vi "Configure Multi Eval Meas Limit ACLR Test Tolerance.vi"(7 "Tolerance 30-40 (5.0)":dbl=5.0 format="%^.3e", 8 "error in (no error)":errorcluster, 9 "Tolerance 23-30 (4.6)":dbl=4.6 format="%^.3e", 10 "Instance (1)":T1=1, 11 "VISA resource name":refnum<visa-resource-name>) -> (0 "error out":errorcluster, 3 "VISA resource name out":refnum<visa-resource-name>)   [LabVIEW 2020, in "Rohde&Schwarz CMXP NR FR2 Measurement.lvlib"]
doc: "Defines the test tolerance for relative ACLR limits, depending on the carrier frequency.\n\nAttribute:\nRSCMXPNRFR2M_ATTR_MULTI_EVAL_MEASUREMENT_LIMIT_ACLR_TEST_TOLERANCE\n\nRemote-control command:\nCONFigure:NRMMw:MEAS<i>:MEValuation:LIMit:ACLR:ATTolerance"
uses:
  <instrlib>/Rohde&Schwarz CMXP NR FR2 Measurement/Rohde&Schwarz CMXP NR FR2 Measurement.lvlib
  <instrlib>/Rohde&Schwarz CMXP NR FR2 Measurement/Private/_Instance.ctl
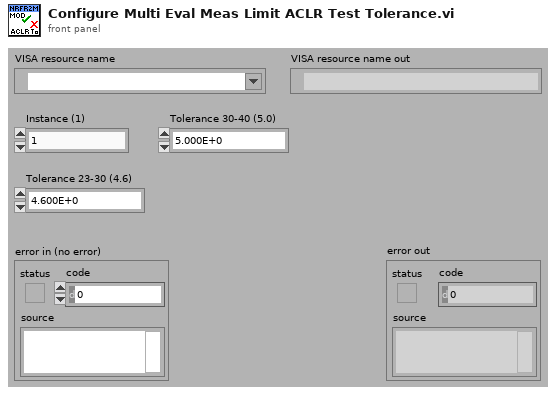
[diagram p1: front panel]
types:
  T1 = typedef "Rohde&Schwarz CMXP NR FR2 Measurement.lvlib/_Instance.ctl" = i32
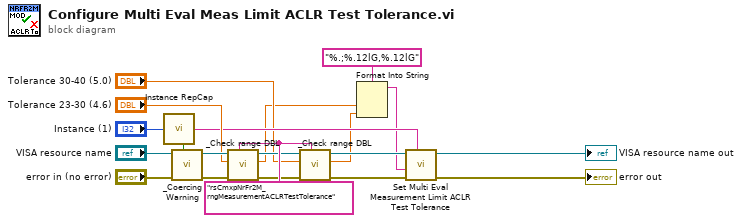
[diagram p0: block diagram]
diagram:
  w17 = "rsCmxpNrFr2M_rngMeasurementACLRTestTolerance"
  n1 = call <instrlib>:"Instance RepCap.vi"("Instance In"="Instance (1)") -> ("In Range?"=w18:bool, "RepCap Identifier Out"=w10:string)  [unwired: 1 in]
  n2 = call <instrlib>:"_Coercing Warning.vi"("In Range?"=w18, "error in (no error)"="error in (no error)", "VISA resource name"="VISA resource name") -> ("error out"=w15:errorcluster, "VISA resource name out"=w16:refnum<visa-resource-name>)  [unwired: 7 in]
  n3 = call <instrlib>:"_Check range DBL.vi"("Range Table Identifier"=w17, "error in (no error)"=w15, "DBL Value In"="Tolerance 23-30 (4.6)", "VISA resource name"=w16) -> ("error out"=w12:errorcluster, "DBL Value Out"=w4:dbl, "VISA resource name out"=w13:refnum<visa-resource-name>)  [unwired: 5 in]
  n4 = call <instrlib>:"_Check range DBL.vi"("Range Table Identifier"=w17, "error in (no error)"=w12, "DBL Value In"="Tolerance 30-40 (5.0)", "VISA resource name"=w13) -> ("error out"=w8:errorcluster, "DBL Value Out"=w3:dbl, "VISA resource name out"=w9:refnum<visa-resource-name>)  [unwired: 5 in]
  n5 = Format Into String(format string="%.;%.12lG,%.12lG", w4, w3) -> (resulting string=w1:string)  [unwired: 2 in, 1 out]
  n6 = call "Set Multi Eval Measurement Limit ACLR Test Tolerance"("Repeated Capabilities"=w10, "error in (no error)"=w8, "Multi Eval Measurement Limit ACLR Test Tolerance ()"=w1, "instrument handle"=w9) -> ("error out"=→"error out":errorcluster, "instrument handle out"=→"VISA resource name out":refnum<visa-resource-name>)  [unwired: 6 in]
